vi "Vision Proc (SubVI).vi"(0 "Image In":T1, 2 "Hue in":i32(knob)=85 scale=0.0..255.0, 3 "Particle Count Limit":i32=10, 5 "Saturation in":i32=110, 6 "Value in":i32=45, 8 "Dilate_its":i32=1, 10 "Image Dst":T1, 11 "Area Size Limit %":dbl=0.10000000000000003, 12 "Score Limits":T2={"Rect Coverage"=55.0, "X Edge Strength"=40.0, "Y Edge Strength"=60.0, "Center"=75.0, "Outer"=75.0, "Vertical"=0.0}, 13 "Margins":cluster{"Hue":i32, "Sat":i32, "Val":i32}={"Hue"=33, "Sat"=53, "Val"=9} {"Sat" scale=0.0..80.0; "Val" scale=0.0..80.0; "Hue" scale=0.0..80.0}, 14 "Erode_its":i32=1, 16 "Camera Type":enum16{"206", "1011"}(ring)=enum."1011", 17 "Annotate":bool=TRUE, 18 "File List":i32(listbox), 19 "Directory":path) -> (20 "Processed Image":T1(plugin-control), 22 "Target Info":T3(array[cluster]), 23 "Value out":cluster{i32, i32}, 25 "Saturation out":cluster{i32, i32}, 26 "Hue":cluster{i32, i32})   [LabVIEW 2015]
uses:
  <vilib>/vision/Image Controls.llb/IMAQ Image.ctl
  <vilib>/vision/NI_Vision_Development_Module.lvlib
panel:
  in  "Image Source":enum32{"File Images", "Live Camera"}(ring)=enum."Live Camera"
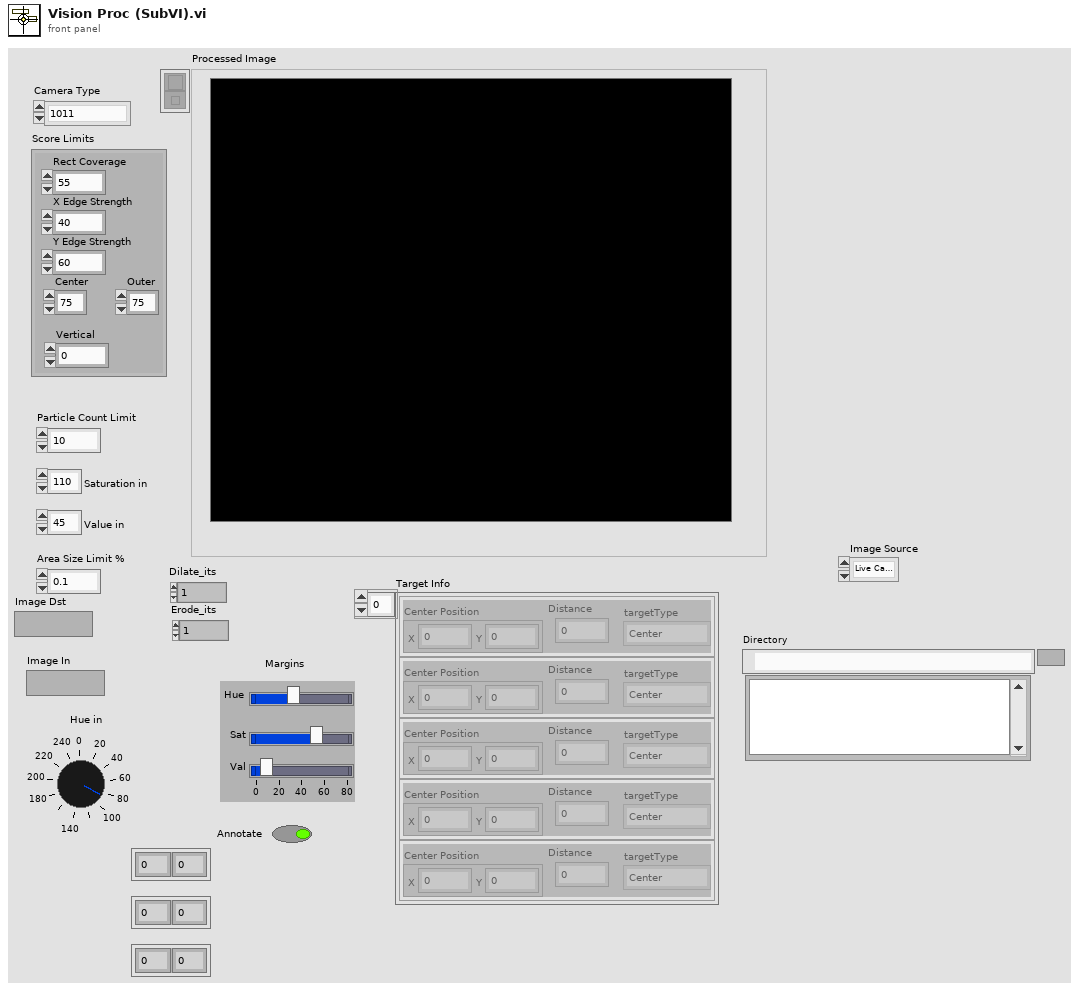
[diagram p1: front panel]
types:
  T1 = typedef "IMAQ Image.ctl" = refnum<image>
  T2 = cluster{"Rect Coverage":dbl, "X Edge Strength":dbl, "Y Edge Strength":dbl, "Center":dbl, "Outer":dbl, "Vertical":dbl}
  T3 = cluster{"Center Position":cluster{"X":dbl, "Y":dbl}, "Distance":dbl, "targetType":enum16{"Center", "Side", "Vertical"}}[]
  T4 = cluster{"Center Position":cluster{"X":dbl, "Y":dbl}, "Distance (ft)":dbl, "targetType":enum16{"Center", "Side", "Vertical"}}[]
  T5 = typedef "Image Type" = u32
  T6 = enum32{"AutoM", "Close", "Dilate", "Erode", "Gradient", "Gradient out", "Gradient in", "Hit miss", "Open", "PClose", "POpen", "Thick", "Thin"}
  T7 = cluster{cluster{"Left":dbl, "Top":dbl, "Right":dbl, "Bottom":dbl}, "Scores":dbl[], cluster{"Long":dbl, "Short":dbl}}[]
  T8 = cluster{"Left":dbl, "Top":dbl, "Right":dbl, "Bottom":dbl}
  T9 = cluster{"Center Position":cluster{"X":dbl, "Y":dbl}, "Distance (ft)":dbl, "targetType":enum16{"Center", "Side", "Vertical"}}
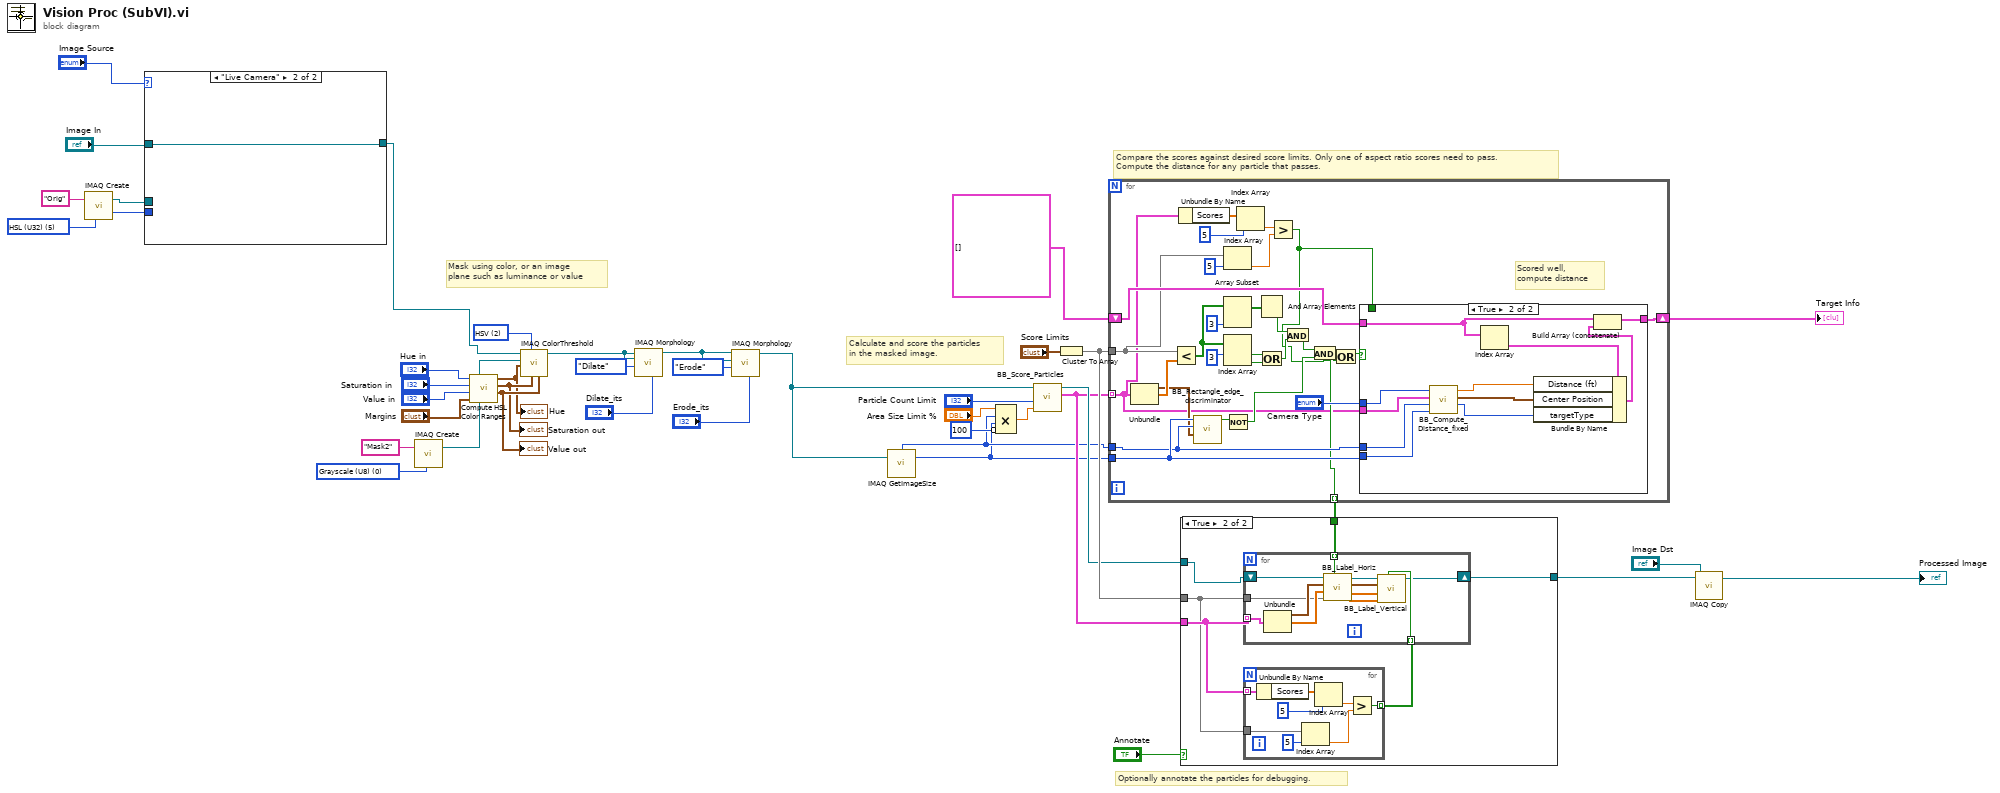
[diagram p0: block diagram]
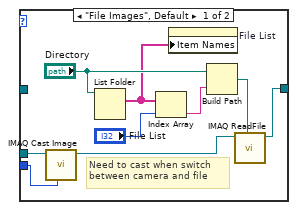
[diagram p2: hidden frame]
diagram:
  w13 = T5 5 items=["Grayscale (U8)", "Grayscale (I16)", "Grayscale (SGL)", "Complex (CSG)", "RGB (U32)", "HSL (U32)", "RGB (U64)", "Grayscale (U16)"] ("Image Type")
  w40 = T5 0 items=["Grayscale (U8)", "Grayscale (I16)", "Grayscale (SGL)", "Complex (CSG)", "RGB (U32)", "HSL (U32)", "RGB (U64)", "Grayscale (U16)"] ("Image Type")
  w32 = u16 2 items=["RGB", "HSL", "HSV", "HSI"] ("Color Mode")
  # "Optionally annotate the particles for debugging."
  # "Compare the scores against desired score limits. Only one of aspect ratio scores need to pass.\nCompute the distance for any particle that passes."
  # "Calculate and score the particles\nin the masked image."
  # "Mask using color, or an image\nplane such as luminance or value"
  n1 = call "IMAQ Create"("Image Name"="Orig", "Image Type"=w13) -> ("New Image"=w12:T1)  [unwired: 2 in, 2 out]
  n2 = case shown="\"Live Camera\"" "Image Source" {
    tunnel: [w44 w51] -> w11
    tunnel: "Image In" -> [_ w51]
    tunnel: w13 -> [w43 _]
    tunnel: w12 -> [w42 _]
    frame "File Images", Default {
      # "Need to cast when switch\nbetween camera and file"
      n3 = call "IMAQ Cast Image"("Image Type"=w43, "Image Src"=w42) -> ("Image Dst Out"=w45:T1)  [unwired: 8 in, 1 out]
      n4 = List Folder(path="Directory") -> (filenames=w46:string[])  [unwired: 3 in, 3 out]
      n5 = Index Array(array=w46, index="File List") -> (element=w49:string)
      n6 = property on="File List" class="LstBox (strict)"("Item Names"=w46) -> ()  [unwired: 2 in, 2 out]
      n7 = Build Path(base path="Directory", name or relative path=w49) -> (appended path=w48:path)
      n8 = call "IMAQ ReadFile"("File Path"=w48, "Image"=w45) -> ("Image Out"=w44:T1)  [unwired: 5 in, 4 out]
    }
    frame "Live Camera" {
    }
  }
  n9 = call "IMAQ Create"("Image Name"="Mask2", "Image Type"=w40) -> ("New Image"=w22:T1)  [unwired: 2 in, 2 out]
  n10 = call "Compute HSL Color Ranges.vi"("Margins"="Margins", "Luminance"="Value in", "Saturation"="Saturation in", "Hue"="Hue in") -> ("Lum Range"=w39:cluster{i32, i32}, "Sat Range"=w38:cluster{i32, i32}, "Hue Range"=w33:cluster{i32, i32})  [unwired: 5 in]
  "Hue" <- w33
  "Saturation out" <- w38
  "Value out" <- w39
  n11 = call "IMAQ ColorThreshold"("Blue or Luma or Val or Inten Range"=w39, "Green or Sat Range"=w38, "Color Mode"=w32, "Red or Hue Range"=w33, "Image Dst"=w22, "Image Src"=w11) -> ("Image Dst Out"=w21:T1)  [unwired: 4 in, 1 out]
  n12 = call "IMAQ Morphology"("Number of iterations (1)"="Dilate_its", "Operation"=T6."Dilate", "Image Dst"=w21, "Image Src"=w21) -> ("Image Dst Out"=w18:T1)  [unwired: 6 in, 1 out]
  n13 = call "IMAQ Morphology"("Number of iterations (1)"="Erode_its", "Operation"=T6."Erode", "Image Dst"=w18, "Image Src"=w18) -> ("Image Dst Out"=w9:T1)  [unwired: 6 in, 1 out]
  n14 = call "IMAQ GetImageSize"("Image"=w9) -> ("Y Resolution"=w6:i32, "X Resolution"=w7:i32)  [unwired: 3 in, 1 out]
  n15 = Compound Arithmetic op=MULTIPLY("Area Size Limit %", w7, w6, invert 100 ("value")) -> (w30:dbl)
  n16 = call "BB_Score_Particles.vi"("Area Size Limit"=w30, "Particle Count Limit"="Particle Count Limit", "Image Refnum in"=w9) -> ("Scored Particle Info"=w8:T7, "Image Refnum out"=w23:T1)  [unwired: 7 in]
  n17 = Cluster To Array(cluster="Score Limits") -> (array=w27:dbl[])
  n18 = for {
    shift-right: [w78] -> w4
    shift-left: T4 [] ("Target Info") -> [w79]
    tunnel: w7 -> [w66]
    tunnel: w8 -> [w59] mode=indexing
    tunnel: w27 -> [w60]
    tunnel: w6 -> [w67]
    tunnel: [w63] -> w28 mode=indexing
    # "Scored well,\ncompute distance"
    n19 = Unbundle(w59) -> (w65:T8, "Scores"=w77:dbl[])  [unwired: 1 out]
    n20 = Less?(x=w60, y=w77) -> (x < y?=w74:bool[])
    n21 = Unbundle By Name(w59) -> ("Scores"=w57:dbl[])
    n22 = call "BB_Rectangle_edge_discriminator.vi"("Cluster"=w65, "X Resolution"=w66, "Y Resolution"=w67) -> ("Edge"=w64:bool)  [unwired: 8 in]
    n23 = Index Array(array=w60, index=5) -> (element=w53:dbl)
    n24 = Array Subset(array=w74, length=3) -> (w75:bool[])  [unwired: 1 in]
    n25 = Index Array(array=w74, index #1=3 ("length")) -> (element #1=w72:bool, element #2=w71:bool)  [unwired: 1 in]
    n26 = Not(x=w64) -> (.not. x?=w61:bool)
    n27 = Index Array(array=w57, index=5) -> (element=w56:dbl)
    n28 = And Array Elements(Boolean array=w75) -> (logical AND=w69:bool)
    n29 = Or(x=w72, y=w71) -> (x .or. y?=w70:bool)
    n30 = Greater?(x=w56, y=w53) -> (0:w52:bool)
    n31 = And(x=w69, y=w70) -> (x .and. y?=w62:bool)
    n32 = And(x=w62, y=w61) -> (x .and. y?=w63:bool)
    n33 = Or(x=w63, y=w52) -> (x .or. y?=w58:bool)
    n34 = case shown="True" w58 {
      tunnel: w79 -> [w80 w86]
      tunnel: [w80 w91] -> w78
      tunnel: w66 -> [_ w90]
      tunnel: "Camera Type" -> [_ w89]
      tunnel: w67 -> [_ w88]
      tunnel: w59 -> [_ w87]
      tunnel: w52 -> [_ _]
      frame False {
        # "Didn't score well enough"
      }
      frame True {
        n35 = call "BB_Compute_Distance_fixed.vi"("Y Image Resolution"=w88, "X Image Resolution"=w90, "Particle Scores"=w87, "Camera Type"=w89) -> ("targetType"=w81:enum16{"Center", "Side", "Vertical"}, "Target Center (-1 to 1)"=w83:cluster{"X":dbl, "Y":dbl}, "Distance (ft)"=w82:dbl)  [unwired: 5 in]
        n36 = Index Array(array=w86) -> (element=w85:T9)  [unwired: 1 in]
        n37 = Bundle By Name(cluster=w85, "Distance (ft)"=w82, "Center Position"=w83, "targetType"=w81) -> (w84:T9)
        n38 = Build Array (concatenate)(w86, w84) -> (w91:T4)
      }
    }
  }
  "Target Info" <- w4
  n39 = case shown="True" "Annotate" {
    tunnel: w23 -> [w92 w93]
    tunnel: [w92 w96] -> w3
    tunnel: w8 -> [_ w97]
    tunnel: w27 -> [_ w94]
    tunnel: w28 -> [_ w98]
    frame False {
    }
    frame True {
      n40 = for {
        tunnel: [w106] -> w95 mode=indexing
        tunnel: w97 -> [w105] mode=indexing
        tunnel: w94 -> [w101]
        n41 = Unbundle By Name(w105) -> ("Scores"=w104:dbl[])
        n42 = Index Array(array=w101, index=5) -> (element=w99:dbl)
        n43 = Index Array(array=w104, index=5) -> (element=w103:dbl)
        n44 = Greater?(x=w103, y=w99) -> (0:w106:bool)
      }
      n45 = for {
        shift-right: [w111] -> w96
        shift-left: w93 -> [w118]
        tunnel: w97 -> [w115] mode=indexing
        tunnel: w94 -> [w114]
        tunnel: w98 -> [w113] mode=indexing
        tunnel: w95 -> [w112] mode=indexing
        n46 = Unbundle(w115) -> (w116:T8, "Scores"=w117:dbl[])  [unwired: 1 out]
        n47 = call "BB_Label_Horiz.vi"("Limit Passed"=w113, "Limits"=w114, "Scores"=w117, "Bounding Box"=w116, "image in"=w118) -> ("Limits Out"=w108:dbl[], "Scores Out"=w109:dbl[], "Bounding BoxOut"=w107:T8, "image out"=w110:T1)  [unwired: 3 in]
        n48 = call "BB_Label_Vertical.vi"("Limit Passed"=w112, "Limits"=w108, "Scores"=w109, "Bounding Box"=w107, "image in"=w110) -> ("image out"=w111:T1)  [unwired: 6 in]
      }
    }
  }
  n49 = call "IMAQ Copy"("Image Dst"="Image Dst", "Image Src"=w3) -> ("Image Dst Out"=→"Processed Image":T1)  [unwired: 4 in, 1 out]
